vi "Station2_QR_Code_correct&localduplication_verification.vi"(9 "BARCODE STATION in":string, 10 "PART_NO":string, 11 "PRIVIOUS code":string[](array[string])) -> (2 "Correct part no True":bool, 3 "Correct part no & No duplication TRUE":bool)   [LabVIEW 2017]
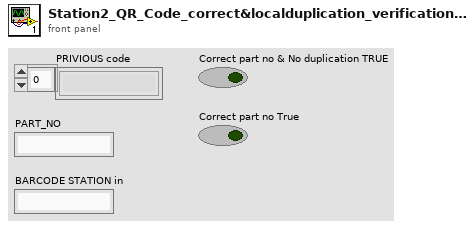
[diagram p1: front panel]
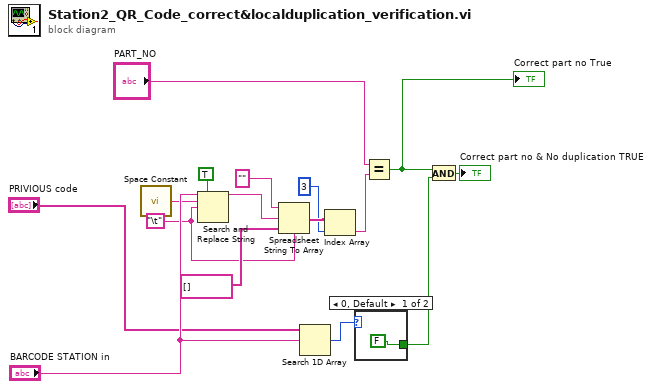
[diagram p0: block diagram]
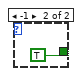
[diagram p2: hidden frame]
diagram:
  w4 = "\t"
  n1 = call <vilib>:"Space Constant.vi"() -> ("String"=w1:string)
  n2 = Search and Replace String(replace all?=TRUE ("replace all? (F)"), input string="BARCODE STATION in", search string=w1, replace string=w4) -> (result string=w3:string)  [unwired: 4 in, 3 out]
  n3 = Spreadsheet String To Array(delimiter (Tab)=w4, format string="", spreadsheet string=w3, array type (2D Dbl)=string[] []) -> (array=w8:string[])
  n4 = Search 1D Array(1D array="PRIVIOUS code", element="BARCODE STATION in") -> (index of element=w13:i32)  [unwired: 1 in]
  n5 = Index Array(array=w8, index=3) -> (element=w9:string)
  n6 = case shown="0, Default" w13 {
    tunnel: [FALSE TRUE] -> w14
    frame 0, Default {
    }
    frame -1 {
    }
  }
  n7 = Equal?(x="PART_NO", y=w9) -> (x = y?=w16:bool)
  "Correct part no True" <- w16
  n8 = And(x=w16, y=w14) -> (x .and. y?=→"Correct part no & No duplication TRUE":bool)
